vi "Regression Equation String.vi"(9 "系数":dbl[](array[numeric]), 10 "精度":i32, 11 "拟合类型":T1(ring)) -> (3 "公式":string)   [LabVIEW 2016, in "曲线模型.xctl"]
doc: "生成回归方程字符串。"
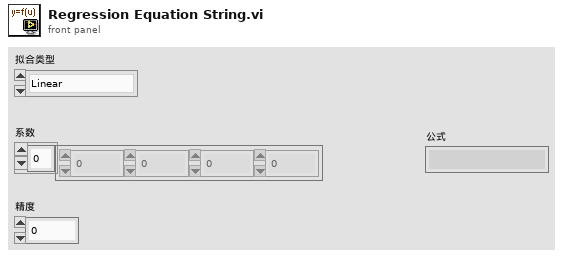
[diagram p1: front panel]
types:
  T1 = enum16{"Linear", "Polynomial", "Exponential", "Power"}
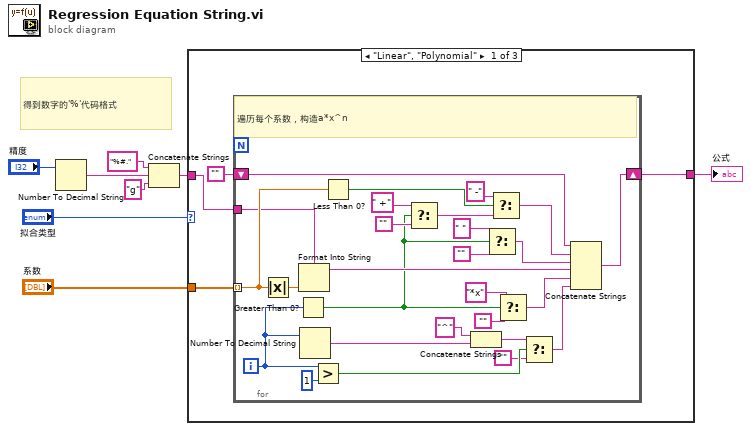
[diagram p0: block diagram]
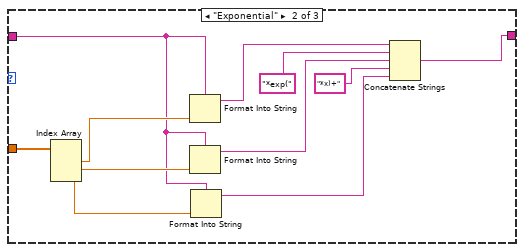
[diagram p2: hidden frame]
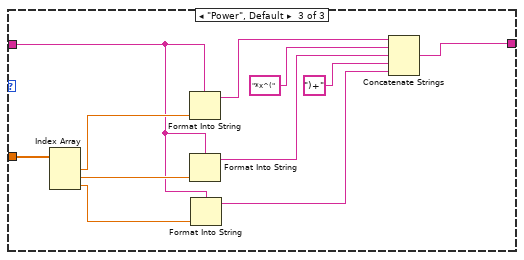
[diagram p3: hidden frame]
diagram:
  # "得到数字的'%'代码格式"
  n1 = Number To Decimal String(number="精度") -> (decimal integer string=w2:string)  [unwired: 1 in]
  n2 = Concatenate Strings("%#." ("format string"), w2, "g" ("format string")) -> (w4:string)
  n3 = case shown="\"Linear\", \"Polynomial\"" "拟合类型" {
    tunnel: [w11 w48 w59] -> w6
    tunnel: "系数" -> [w12 w47 w58]
    tunnel: w4 -> [w9 w42 w53]
    frame "Linear", "Polynomial" {
      n4 = for {
        tunnel: w12 -> [w39] mode=indexing
        shift-right: [w27] -> w11
        shift-left: "" -> [w28]
        tunnel: w9 -> [w18]
        i -> [w34]
        # "遍历每个系数，构造a*x^n"
        n5 = Absolute Value(x=w39) -> (abs(x)=w20:dbl)
        n6 = Greater Than 0?(x=w34) -> (x > 0?=w13:bool)
        n7 = Format Into String(format string=w18, w20) -> (resulting string=w19:string)  [unwired: 2 in, 1 out]
        n8 = Number To Decimal String(number=w34) -> (decimal integer string=w30:string)  [unwired: 1 in]
        n9 = Greater?(x=w34, y=1) -> (0:w32:bool)
        n10 = Less Than 0?(x=w39) -> (x < 0?=w38:bool)
        n11 = Select(t=" +", s=w13, f="") -> (s? t:f=w14:string)
        n12 = Concatenate Strings("^", w30) -> (w22:string)
        n13 = Select(t=" ", s=w13, f="") -> (s? t:f=w25:string)
        n14 = Select(t=" -", s=w38, f=w14) -> (s? t:f=w26:string)
        n15 = Select(t="*x", s=w13, f="") -> (s? t:f=w24:string)
        n16 = Select(t=w22, s=w32, f="") -> (s? t:f=w23:string)
        n17 = Concatenate Strings(w28, w26, w25, w19, w24, w23) -> (w27:string)
      }
    }
    frame "Exponential" {
      n18 = Index Array(array=w47) -> (element #1=w46:dbl, element #2=w44:dbl, element #3=w41:dbl)  [unwired: 3 in]
      n19 = Format Into String(format string=w42, w46) -> (resulting string=w45:string)  [unwired: 2 in, 1 out]
      n20 = Format Into String(format string=w42, w44) -> (resulting string=w43:string)  [unwired: 2 in, 1 out]
      n21 = Format Into String(format string=w42, w41) -> (resulting string=w40:string)  [unwired: 2 in, 1 out]
      n22 = Concatenate Strings(w45, "*exp(", w43, "*x)+", w40) -> (w48:string)
    }
    frame "Power", Default {
      n23 = Index Array(array=w58) -> (element #1=w57:dbl, element #2=w55:dbl, element #3=w52:dbl)  [unwired: 3 in]
      n24 = Format Into String(format string=w53, w57) -> (resulting string=w56:string)  [unwired: 2 in, 1 out]
      n25 = Format Into String(format string=w53, w55) -> (resulting string=w54:string)  [unwired: 2 in, 1 out]
      n26 = Format Into String(format string=w53, w52) -> (resulting string=w51:string)  [unwired: 2 in, 1 out]
      n27 = Concatenate Strings(w56, "*x^(", w54, ")+", w51) -> (w59:string)
    }
  }
  "公式" <- w6
